vi "PlaceNewTarget.vi"(8 "error in (no error)":errorcluster, 11 "Game Data in":T1) -> (0 "error out":errorcluster, 3 "Game Data out":T1)   [LabVIEW 2020]
doc: "This VI finds empty spaces on a board and chooses one at random.\nIf none is found returns (-1,-1)"
uses:
  TypeDef/game-data.ctl
  TypeDef/tiles-key.ctl
  <vilib>/numeric/Random Number (Range) I64.vi
  <vilib>/numeric/sub_Random U32.vi
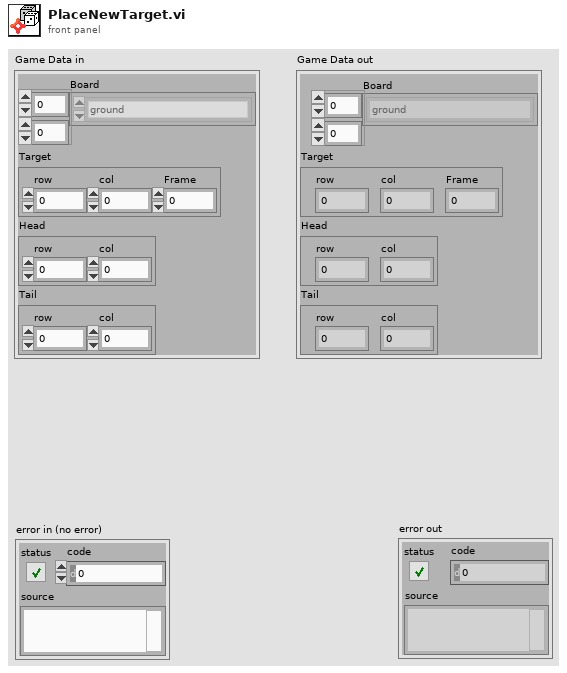
[diagram p1: front panel]
types:
  T1 = typedef "game-data.ctl" = cluster{"Board":T2[][], "Target":cluster{"row":i32, "col":i32, "Frame":i8}, "Head":cluster{"row":i32, "col":i32}, "Tail":cluster{"row":i32, "col":i32}}
  T2 = typedef "tiles-key.ctl" = enum16{"ground", "wall", "head (right)", "head (up)", "head (left)", "head (down)", "L-turn (right-up)", "L-turn (up-left)", "L-turn (left-down)", "L-turn (down-right)", "body (right)", "body (up)", "body (left)", "body (down)", "R-turn (right-down)", "R-turn (up-right)", "R-turn (left-up)", "R-turn (down-left)", "tail (right)", "tail (up)", "tail (left)", "tail (down)", "dead head (right)", "dead head (up)", "dead head (left)", "dead head (down)", "dead L-turn (right-up)", "dead L-turn (up-left)", "dead L-turn (left-down)", "dead L-turn (down-right)", "dead body (right)", "dead body (up)", "dead body (left)", "dead body (down)", "dead R-turn (right-down)", "dead R-turn (up-right)", "dead R-turn (left-up)", "dead R-turn (down-left)", "dead tail (right)", "dead tail (up)", "dead tail (left)", "dead tail (down)", "target red", "target blue", "target yellow", "target green"}
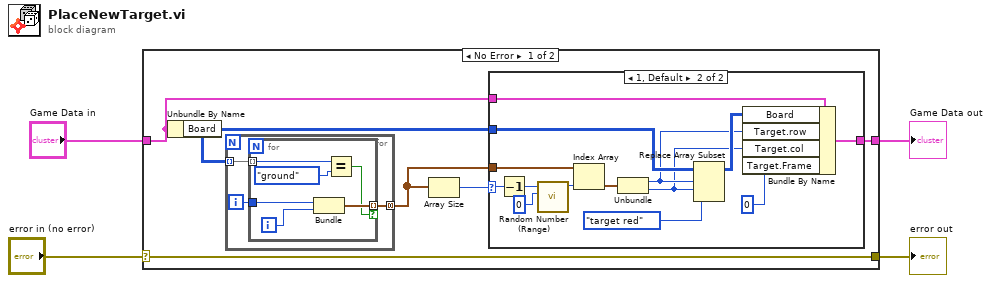
[diagram p0: block diagram]
diagram:
  n1 = case shown="No Error" "error in (no error)" {
    selector: "error in (no error)" -> [w10 w36]
    tunnel: [w10 w36] -> w3
    tunnel: "Game Data in" -> [w6 w35]
    tunnel: [w5 w35] -> w1
    frame No Error {
      n2 = Unbundle By Name(w6) -> ("Board"=w7:T2[][])
      n3 = for {
        tunnel: w7 -> [w28] mode=indexing
        tunnel: [w26] -> w9 mode=concatenating
        i -> [w27]
        n4 = for {
          tunnel: w28 -> [w34] mode=indexing
          tunnel: w27 -> [w30]
          tunnel: [w32] -> w26 mode=indexing if=w31
          i -> [w29]
          n5 = Bundle(w30, w29) -> (w32:cluster{i32, i32})  [unwired: 1 in]
          n6 = Equal?(x=w34, y=tiles-key."ground") -> (x = y?=w31:bool)
        }
      }
      n7 = Array Size(array=w9) -> (size(s)=w8:i32)
      n8 = case shown="1, Default" w8 {
        selector: w8 -> [_ w21]
        tunnel: w9 -> [_ w24]
        tunnel: w7 -> [_ w19]
        tunnel: w6 -> [w11 w17]
        tunnel: [w11 w12] -> w5
        frame 0 {
        }
        frame 1, Default {
          n9 = Decrement(x=w21) -> (x-1=w25:i32)
          n10 = call-poly <vilib>:"Random Number (Range).vi"("lower bound (-100)"=i64 0, "upper bound (100)"=w25) -> ("number"=w23:i64)  [unwired: 9 in]
          n11 = Index Array(array=w24, index=w23) -> (element=w22:cluster{i32, i32})
          n12 = Unbundle(w22) -> (w15:i32, w14:i32)
          n13 = Replace Array Subset(array=w19, new element=tiles-key."target red" ("new element/subarray"), index (row)=w15, index (col)=w14) -> (w16:T2[][])
          n14 = Bundle By Name(cluster=w17, "Board"=w16, "Target.row"=w15, "Target.col"=w14, "Target.Frame"=i8 0) -> (w12:T1)
        }
      }
    }
    frame Error {
    }
  }
  "error out" <- w3
  "Game Data out" <- w1
